vi "EXCOM-INI.vi"(0 "TCS VRN IN":refnum<visa-resource-name>, 9 "Port Number":i32) -> (4 "TCS VRN OUT":refnum<visa-resource-name>, 15 "error out":errorcluster)   [LabVIEW 2011]
uses:
  <vilib>/Instr/_visa.llb/VISA Configure Serial Port (Instr).vi
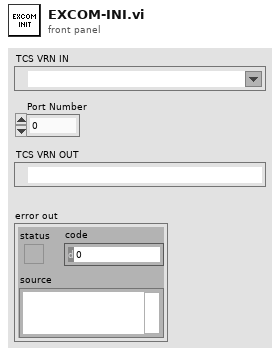
[diagram p1: front panel]
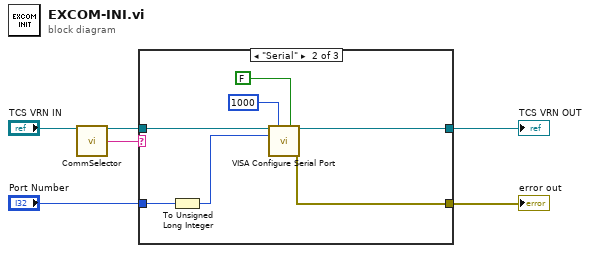
[diagram p0: block diagram]
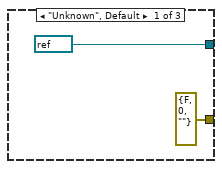
[diagram p2: hidden frame]
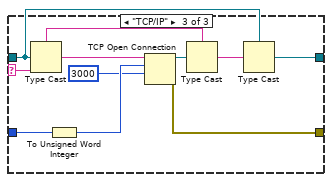
[diagram p3: hidden frame]
diagram:
  n1 = call "CommSelector.vi"("VISA resource name"="TCS VRN IN") -> ("VISA resource name"=w3:refnum<visa-resource-name>, "CommType"=w5:string)  [unwired: 13 in]
  n2 = case shown="\"Serial\"" w5 {
    selector: w5 -> [_ _ w20]
    tunnel: "Port Number" -> [_ w14 w24]
    tunnel: w3 -> [_ w15 w19]
    tunnel: [refnum<visa-resource-name> "-1" ("VISA resource name") w12 w17] -> w2
    tunnel: [errorcluster {"status"=FALSE, "code"=0, "source"=""} ("error out") w10 w16] -> w1
    frame "Unknown", Default {
    }
    frame "Serial" {
      n3 = To Unsigned Long Integer(number=w14) -> (unsigned 32bit integer=w11:u32)
      n4 = call-poly "VISA Configure Serial Port"("VISA resource name"=w15, "timeout (10sec)"=u32 1000, "Enable Termination\nChar (T)"=FALSE ("Enable Termination\nChar (T)"), "baud rate (9600)"=w11) -> ("VISA resource name out"=w12:refnum<visa-resource-name>, "error out"=w10:errorcluster)  [unwired: 10 in]
    }
    frame "TCP/IP" {
      n5 = Type Cast(type=w20, x=w19) -> (*(type *) &x=w25:string)
      n6 = To Unsigned Word Integer(number=w24) -> (unsigned 16bit integer=w23:u16)
      n7 = TCP Open Connection(address=w25, remote port or service name=w23, timeout ms (60000)=3000) -> (connection ID=w21:refnum<k5>, error out=w16:errorcluster)  [unwired: 2 in]
      n8 = Type Cast(type=w20, x=w21) -> (*(type *) &x=w18:string)
      n9 = Type Cast(type=w19, x=w18) -> (*(type *) &x=w17:refnum<visa-resource-name>)
    }
  }
  "TCS VRN OUT" <- w2
  "error out" <- w1
